vi "Write Variant recursive.vi"(8 "error in (no error)":errorcluster, 9 "Section":string[](array[string]), 10 "Value Cluster in":variant, 11 "Root Node":variant) -> (0 "error out":errorcluster, 3 "Root Node out":variant)   [LabVIEW 2020, in "hse-config.lvlib" / "config-base.lvclass"]
doc: "____\nHAMPEL SOFTWARE ENGINEERING v3.8.0 (2023-12-18 14:41)"
uses:
  config-base.lvclass
  hse-misc/Type_Descriptor/TypeDescriptor_GetPString.vi
  config-base.lvclass/config-base.ctl
  <vilib>/Utility/Data Type/NI_Data Type.lvlib
  hse-misc/hse-misc.lvlib
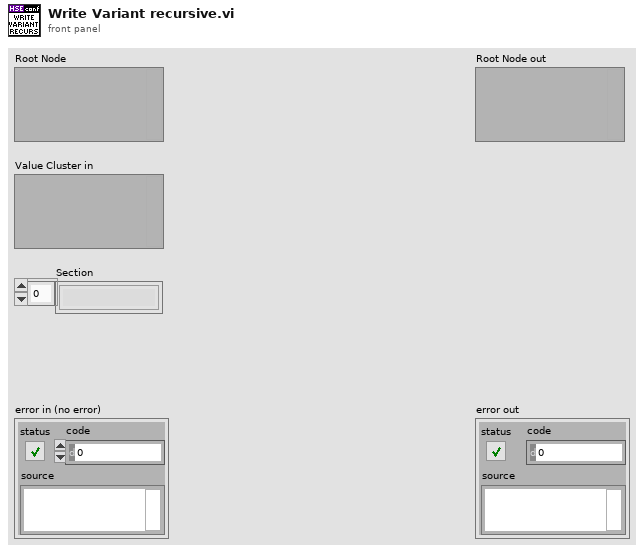
[diagram p1: front panel]
types:
  T1 = typedef "NI_Data Type.lvlib/Data Type.ctl" = enum8{"Invalid Type", "Void", "I8", "I16", "I32", "I64", "U8", "U16", "U32", "U64", "Single Float", "Double Float", "Extended Float", "Single Complex", "Double Complex", "Extended Complex", "Enum U8", "Enum U16", "Enum U32", "Enum U64", "Single Float With Unit", "Double Float With Unit", "Extended Float With Unit", "Single Complex with Unit", "Double Complex with Unit", "Extended Complex with Unit", "Boolean", "String", "Path", "Picture", "Tag", "Array", "Cluster", "Variant", "LV Variant", "Waveform", "Timestamp", "Digital Waveform", "Digital Data", "ExpressData", "Refnum", "External Data", "VI", "Poly VI", "LabVIEW Class Instance", "Fixed Point", "Set Collection", "Map Collection"}
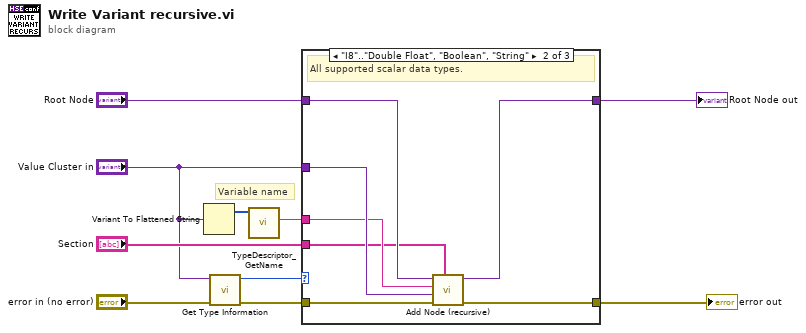
[diagram p0: block diagram]
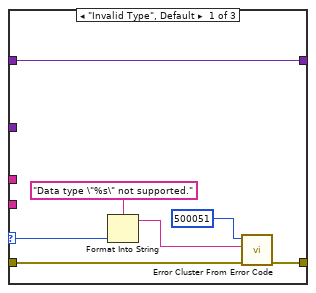
[diagram p2: hidden frame]
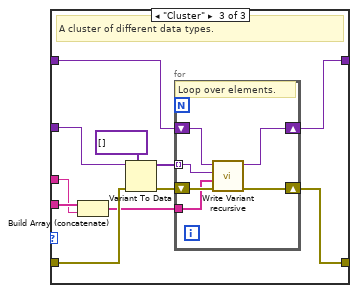
[diagram p3: hidden frame]
diagram:
  # "Variable name"
  n1 = Variant To Flattened String(Variant="Value Cluster in") -> (1:w9:i16[])  [unwired: 1 out]
  n2 = call <vilib>:"Get Type Information.vi"("error in (no error)"="error in (no error)", "variant"="Value Cluster in") -> ("error out"=w8:errorcluster, "type"=w7:T1)  [unwired: 5 in, 3 out]
  n3 = call "TypeDescriptor_GetName.vi"("type descriptor"=w9) -> ("name"=w10:string)  [unwired: 8 in, 2 out]
  n4 = case shown="\"I8\"..\"Double Float\", \"Boolean\", \"String\"" w7 {
    selector: w7 -> [w13 _ _]
    tunnel: w8 -> [w14 w24 w31]
    tunnel: [w12 w23 w25] -> w5
    tunnel: "Value Cluster in" -> [_ w22 w32]
    tunnel: w10 -> [_ w20 w34]
    tunnel: "Root Node" -> [w11 w21 w28]
    tunnel: [w11 w19 w26] -> w4
    tunnel: "Section" -> [_ w18 w35]
    frame "Invalid Type", Default {
      n5 = Format Into String(format string="Data type \"%s\" not supported.", w13) -> (resulting string=w16:string)  [unwired: 2 in, 1 out]
      n6 = call <vilib>:"Error Cluster From Error Code.vi"("error in (no error)"=w14, "error message (\"\")"=w16, "error code (0)"=500051) -> ("error out"=w12:errorcluster)  [unwired: 6 in]
    }
    frame "I8".."Double Float", "Boolean", "String" {
      # "All supported scalar data types."
      n7 = call "Add Node (recursive).vi"("Section"=w18, "error in"=w24, "Value"=w22, "Key"=w20, "Node in"=w21) -> ("error out"=w23:errorcluster, "Node out"=w19:variant)  [unwired: 5 in]
    }
    frame "Cluster" {
      # "A cluster of different data types."
      n8 = Build Array (concatenate)(w35, w34) -> (w27:string[])
      n9 = Variant To Data(error in=w31, type=variant[] [], Variant=w32) -> (data=w29:variant[], error out=w30:errorcluster)
      n10 = for {
        tunnel: w29 -> [w39] mode=indexing
        tunnel: w27 -> [w38]
        shift-right: [w37] -> w25
        shift-left: w30 -> [w41]
        shift-right: [w36] -> w26
        shift-left: w28 -> [w40]
        # "Loop over elements."
        n11 = call "Write Variant recursive.vi"("error in (no error)"=w41, "Section"=w38, "Value Cluster in"=w39, "Root Node"=w40) -> ("error out"=w37:errorcluster, "Root Node out"=w36:variant)  [unwired: 6 in]
      }
    }
  }
  "error out" <- w5
  "Root Node out" <- w4
